vi "prepareToNoAck.vi"(6 "iteration":i32, 8 "error in (no error)":errorcluster, 9 "lostCmdId":i32, 10 "cmd":string, 11 "tcpServerCmd in":refnum<class "TcpServerCmd.lvclass">) -> (0 "error out":errorcluster, 2 "JSON string":string, 3 "tcpServerCmd out":refnum<class "TcpServerCmd.lvclass">)   [LabVIEW 2018, in "TcpServerCmd.lvclass"]
doc: "Prepare the command received to send the noAck to TCP Client."
uses:
  TcpServerCmd.lvclass
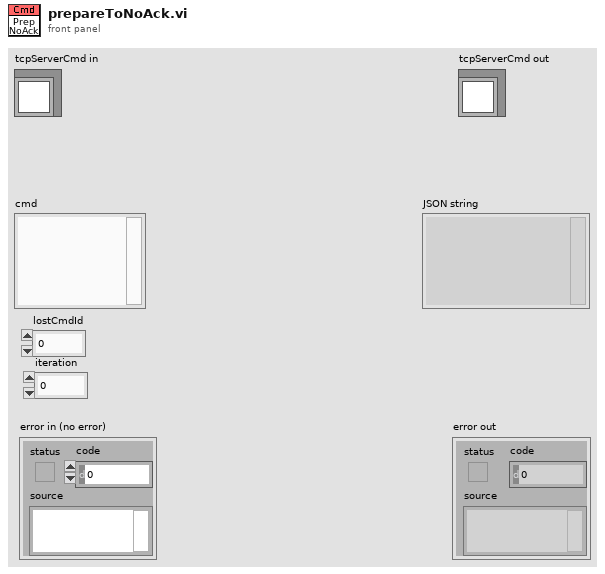
[diagram p1: front panel]
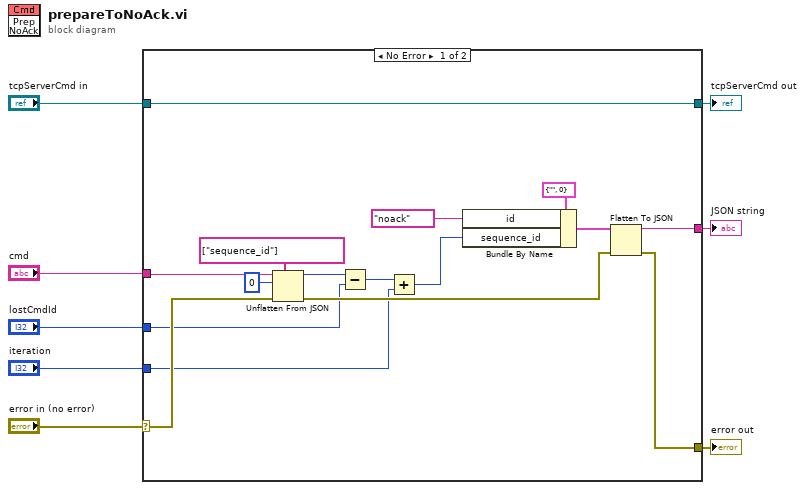
[diagram p0: block diagram]
diagram:
  n1 = case shown="No Error" "error in (no error)" {
    selector: "error in (no error)" -> [w19 w26]
    tunnel: [w17 w26] -> w7
    tunnel: [w24 w25] -> w5
    tunnel: "tcpServerCmd in" -> [w24 w25]
    tunnel: "cmd" -> [w10 _]
    tunnel: [w20 _] -> w3
    tunnel: "lostCmdId" -> [w13 _]
    tunnel: "iteration" -> [w15 _]
    frame No Error {
      n2 = Unflatten From JSON(path=string[] ["sequence_id"], JSON string=w10, type and defaults=0, error in (no error)=w19) -> (value=w14:i32, error out=w18:errorcluster)  [unwired: 3 in]
      n3 = Subtract(x=w14, y=w13) -> (x-y=w12:i32)
      n4 = Add(x=w12, y=w15) -> (x+y=w16:i32)
      n5 = Bundle By Name(cluster=cluster{"id":string, "sequence_id":i32} {"id"="", "sequence_id"=0}, "id"="noack" ("cmdStatus"), "sequence_id"=w16) -> (w21:cluster{"id":string, "sequence_id":i32})
      n6 = Flatten To JSON(anything=w21, error in (no error)=w18) -> (JSON string=w20:string, 11:w17:errorcluster)  [unwired: 1 in]
    }
    frame Error {
    }
  }
  "error out" <- w7
  "tcpServerCmd out" <- w5
  "JSON string" <- w3
